vi "Pre Launch Init.vi"(11 "UserManagement In":refnum<class "UserManagement.lvclass">) -> (0 "Error Out":errorcluster, 3 "UserManagement Out":refnum<class "UserManagement.lvclass">)   [LabVIEW 2019, in "UserManagement.lvlib" / "UserManagement.lvclass"]
uses:
  UserManagement.lvclass
  UserManagement.lvclass/UserManagement.ctl
  <vilib>/NI/Event Source Actor/Event Source/Event Source/Event Source.lvclass
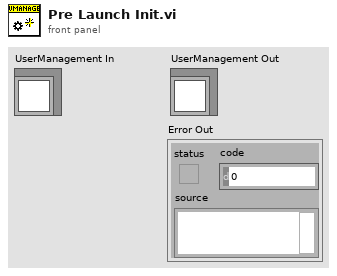
[diagram p1: front panel]
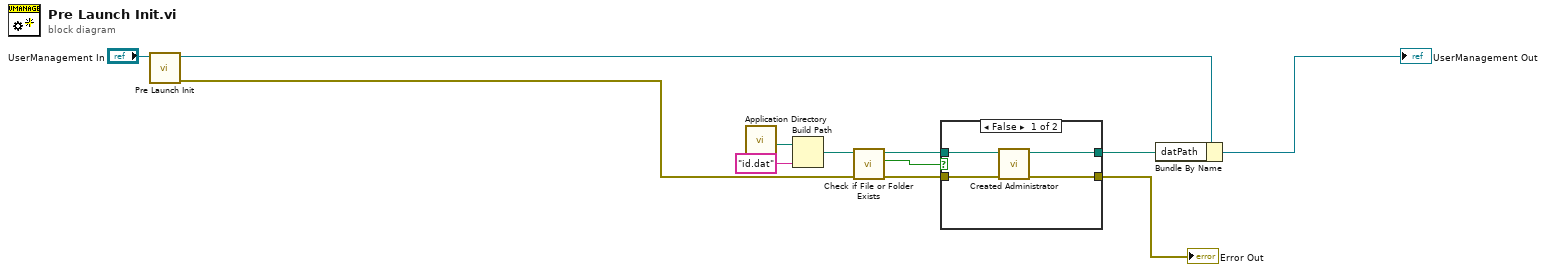
[diagram p0: block diagram]
diagram:
  n1 = call-parent "Pre Launch Init.vi"("Event Source In"="UserManagement In") -> ("Error Out"=w6:errorcluster, "Event Source Out"=w9:refnum<class "UserManagement.lvclass">)  [unwired: 9 in]
  n2 = call <vilib>:"Application Directory.vi"() -> ("Application Directory"=w11:path)
  n3 = Build Path(base path=w11, name or relative path="id.dat") -> (appended path=w7:path)
  n4 = call <vilib>:"Check if File or Folder Exists.vi"("error in (no error)"=w6, "path"=w7) -> ("error out"=w3:errorcluster, "file or folder exists?"=w5:bool, "dup path"=w4:path)  [unwired: 7 in]
  n5 = case shown="False" w5 {
    tunnel: w4 -> [w16 w18]
    tunnel: w3 -> [w15 w17]
    tunnel: [w14 w18] -> w2
    tunnel: [w13 w17] -> w1
    frame False {
      n6 = call "Created Administrator.vi"("error in (no error)"=w15, "File Path Control"=w16) -> ("error out"=w13:errorcluster, "File Path out"=w14:path)  [unwired: 8 in]
    }
    frame True {
    }
  }
  "Error Out" <- w1
  n7 = Bundle By Name(cluster=w9, "datPath"=w2) -> (→"UserManagement Out":refnum<class "UserManagement.lvclass">)
